vi "system to string.vi"(8 "error in":errorcluster, 11 "system":T1) -> (0 "error out":errorcluster, 2 "data":string)   [LabVIEW 2013, in "PLConfigurationSerializer.lvlib"]
uses:
  PLConfigurationSerializer.lvlib
  systems cluster.ctl
  system configuration/PL_System Configuration.lvclass
  targets cluster.ctl
  target configuration/PL_Target Configuration.lvclass
  engines cluster.ctl
  <vilib>/NI/Module Execution Interface/Engine Configuration/engine configuration.lvclass
  <vilib>/NI/Tag Bus Module Framework/module configuration/TBM module configuration.lvclass
  targetlist.ctl
  target configuration/PL_Target Configuration.lvclass/PL_Target Configuration.ctl
  enginelist.ctl
  modulelist.ctl
  <vilib>/NI/Tag Bus Module Framework/root configuration/TBM configuration.lvclass/TBM configuration.ctl
  <vilib>/NI/Tag Bus Module Framework/root configuration/create GUID.vi
  <vilib>/NI/Tag Bus Module Framework/root configuration/TBM configuration.lvclass
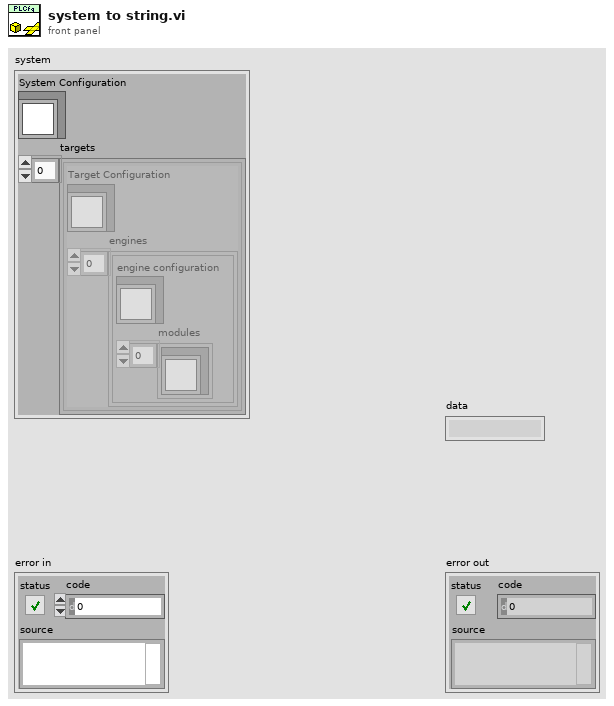
[diagram p1: front panel]
types:
  T1 = typedef "PLConfigurationSerializer.lvlib/systems cluster.ctl" = cluster{"System Configuration":refnum<class "PL_System Configuration.lvclass">, "targets":T2[]}
  T2 = typedef "PLConfigurationSerializer.lvlib/targets cluster.ctl" = cluster{"Target Configuration":refnum<class "PL_Target Configuration.lvclass">, "engines":T3[]}
  T3 = typedef "PLConfigurationSerializer.lvlib/engines cluster.ctl" = cluster{"engine configuration":refnum<class "engine configuration.lvclass">, "modules":refnum<class "TBM module configuration.lvclass">[]}
  T4 = typedef "PLConfigurationSerializer.lvlib/targetlist.ctl" = cluster{"name":string, "instanceid":string}
  T5 = typedef "PLConfigurationSerializer.lvlib/enginelist.ctl" = cluster{"engineid":string, "classname":string}
  T6 = typedef "PLConfigurationSerializer.lvlib/modulelist.ctl" = cluster{"moduleid":string, "classname":string}
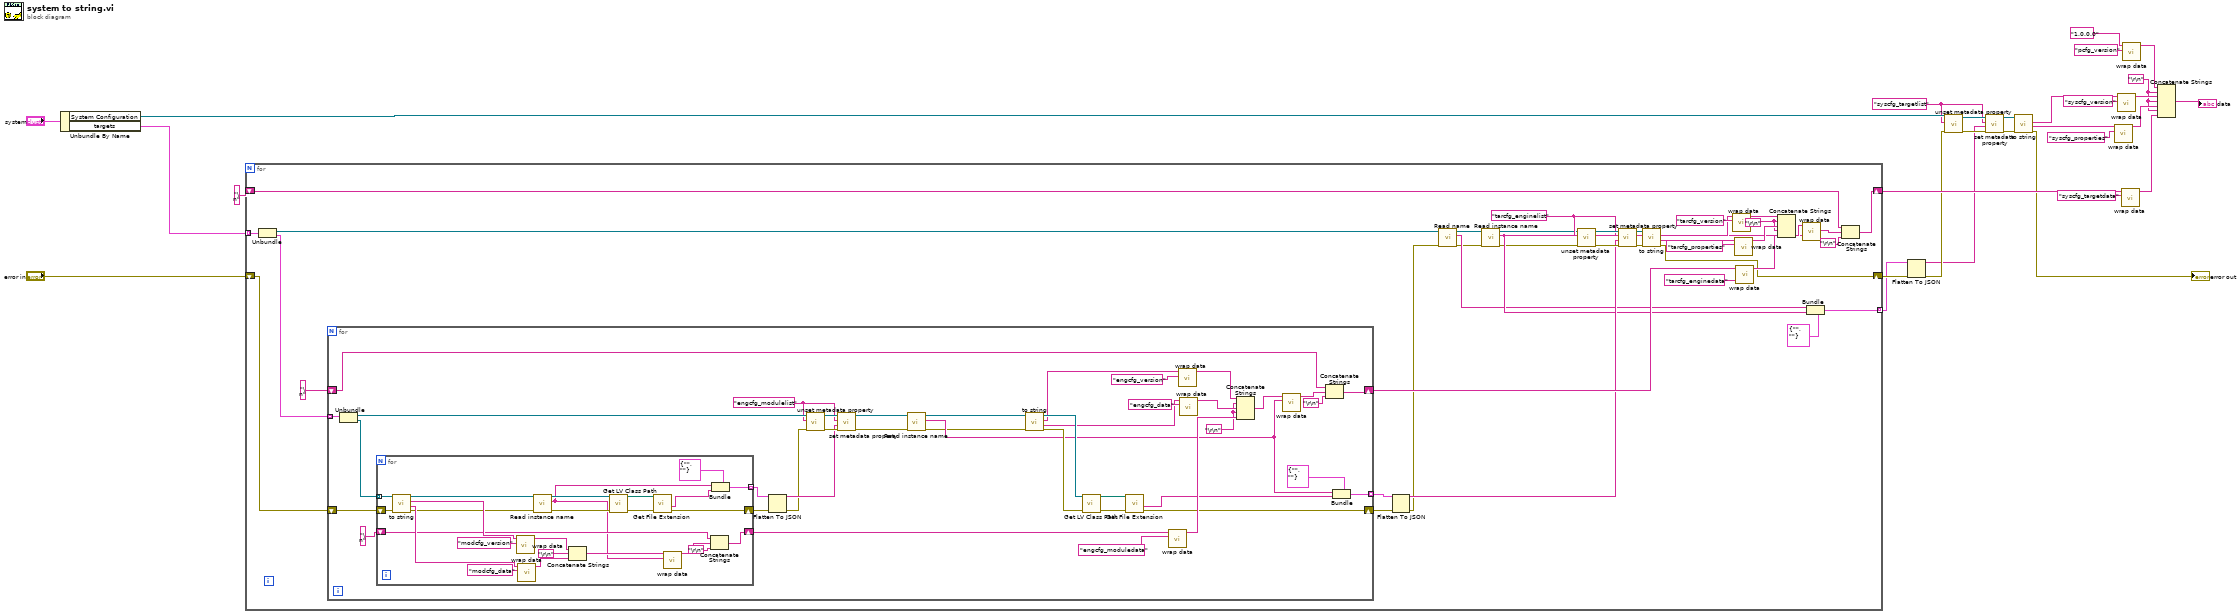
[diagram p0: block diagram]
diagram:
  w2 = "syscfg_targetlist" ("additional identifier")
  w16 = "\r\n"
  n1 = Unbundle By Name("system") -> ("System Configuration"=w7:refnum<class "PL_System Configuration.lvclass">, "targets"=w23:T2[])
  n2 = for {
    tunnel: w23 -> [w67] mode=indexing
    shift-right: [w47] -> w11
    shift-left: "error in" -> [w48]
    shift-right: [w60] -> w19
    shift-left: "\n" -> [w59]
    tunnel: [w44] -> w10 mode=indexing
    w41 = "tarcfg_enginelist" ("additional identifier")
    w52 = "\r\n"
    n3 = Unbundle(w67) -> ("Target Configuration"=w33:refnum<class "PL_Target Configuration.lvclass">, "engines"=w55:T3[])
    n4 = for {
      shift-right: [w75] -> w39
      shift-left: w48 -> [w84]
      tunnel: w55 -> [w107] mode=indexing
      shift-right: [w98] -> w50
      shift-left: "\n" -> [w97]
      tunnel: [w92] -> w40 mode=indexing
      w79 = "engcfg_modulelist" ("additional identifier")
      w87 = "\r\n"
      n5 = Unbundle(w107) -> ("engine configuration"=w80:refnum<class "engine configuration.lvclass">, "modules"=w106:refnum<class "TBM module configuration.lvclass">[])
      n6 = for {
        tunnel: w106 -> [w131] mode=indexing
        shift-right: [w111] -> w86
        shift-left: w84 -> [w132]
        shift-right: [w120] -> w100
        shift-left: "\n" -> [w118]
        tunnel: [w117] -> w83 mode=indexing
        n7 = call-dynamic "to string.vi"("error in"=w132, "module configuration in"=w131) -> ("error out"=w108:errorcluster, "data"=w127:string, "version"=w130:string, "module configuration out"=w122:refnum<class "TBM module configuration.lvclass">)  [unwired: 6 in]
        n8 = call <vilib>:"wrap data.vi"("identifier"="modcfg_version" ("additional identifier"), "data to wrap"=w130) -> ("wrapped data"=w124:string)  [unwired: 9 in]
        n9 = call <vilib>:"wrap data.vi"("identifier"="modcfg_data" ("additional identifier"), "data to wrap"=w127) -> ("wrapped data"=w126:string)  [unwired: 9 in]
        n10 = call <vilib>:"Read instance name.vi"("error in"=w108, "configuration in"=w122) -> ("error out"=w110:errorcluster, "instance id"=w109:string, "configuration out"=w112:refnum<class "TBM module configuration.lvclass">)  [unwired: 7 in]
        n11 = Concatenate Strings(w124, "\r\n", w126) -> (w123:string)
        n12 = call <vilib>:"Get LV Class Path.vi"("error in (no error)"=w110, "object"=w112) -> ("error out"=w114:errorcluster, "class path"=w115:path)  [unwired: 8 in]
        n13 = call <vilib>:"Get File Extension.vi"("error in (no error)"=w114, "file"=w115) -> ("error out"=w111:errorcluster, "filename without extension"=w113:string)  [unwired: 6 in, 2 out]
        n14 = call <vilib>:"wrap data.vi"("identifier"=w109, "data to wrap"=w123) -> ("wrapped data"=w119:string)  [unwired: 9 in]
        n15 = Concatenate Strings(w118, w119, "\r\n") -> (w120:string)
        n16 = Bundle(cluster=T6 {"moduleid"="", "classname"=""} ("modulelist"), "moduleid"=w109, "classname"=w113) -> (w117:T6)
      }
      n17 = Flatten To JSON(anything=w83, error in (no error)=w86) -> (JSON string=w78:string, 11:w77:errorcluster)  [unwired: 1 in]
      n18 = call <vilib>:"unset metadata property.vi"("error in"=w77, "key"=w79, "configuration in"=w80) -> ("error out"=w82:errorcluster, "configuration out"=w81:refnum<class "engine configuration.lvclass">)  [unwired: 7 in]
      n19 = call <vilib>:"set metadata property.vi"("error in"=w82, "value"=w78, "key"=w79, "configuration in"=w81) -> ("error out"=w68:errorcluster, "configuration out"=w69:refnum<class "engine configuration.lvclass">)  [unwired: 6 in]
      n20 = call <vilib>:"Read instance name.vi"("error in"=w68, "configuration in"=w69) -> ("error out"=w71:errorcluster, "instance id"=w72:string, "configuration out"=w70:refnum<class "engine configuration.lvclass">)  [unwired: 7 in]
      n21 = call-dynamic "to string.vi"("error in"=w71, "engine configuration in"=w70) -> ("error out"=w105:errorcluster, "data"=w93:string, "version"=w94:string, "engine configuration out"=w95:refnum<class "engine configuration.lvclass">)  [unwired: 6 in]
      n22 = call <vilib>:"Get LV Class Path.vi"("error in (no error)"=w105, "object"=w95) -> ("error out"=w76:errorcluster, "class path"=w74:path)  [unwired: 8 in]
      n23 = call <vilib>:"Get File Extension.vi"("error in (no error)"=w76, "file"=w74) -> ("error out"=w75:errorcluster, "filename without extension"=w73:string)  [unwired: 6 in, 2 out]
      n24 = call <vilib>:"wrap data.vi"("identifier"="engcfg_moduledata" ("additional identifier"), "data to wrap"=w100) -> ("wrapped data"=w89:string)  [unwired: 9 in]
      n25 = call <vilib>:"wrap data.vi"("identifier"="engcfg_version" ("additional identifier"), "data to wrap"=w94) -> ("wrapped data"=w91:string)  [unwired: 9 in]
      n26 = call <vilib>:"wrap data.vi"("identifier"="engcfg_data" ("additional identifier"), "data to wrap"=w93) -> ("wrapped data"=w90:string)  [unwired: 9 in]
      n27 = Concatenate Strings(w91, w87, w90, w87, w89) -> (w88:string)
      n28 = call <vilib>:"wrap data.vi"("identifier"=w72, "data to wrap"=w88) -> ("wrapped data"=w96:string)  [unwired: 9 in]
      n29 = Concatenate Strings(w97, w96, "\r\n") -> (w98:string)
      n30 = Bundle(cluster=T5 {"engineid"="", "classname"=""} ("enginelist"), "engineid"=w72, "classname"=w73) -> (w92:T5)
    }
    n31 = Flatten To JSON(anything=w40, error in (no error)=w39) -> (JSON string=w38:string, 11:w32:errorcluster)  [unwired: 1 in]
    n32 = call "Read name.vi"("error in"=w32, "PL_Local Target Configuration in"=w33) -> ("error out"=w31:errorcluster, "name"=w36:string, "PL_Local Target Configuration out"=w34:refnum<class "PL_Target Configuration.lvclass">)  [unwired: 7 in]
    n33 = call <vilib>:"Read instance name.vi"("error in"=w31, "configuration in"=w34) -> ("error out"=w30:errorcluster, "instance id"=w37:string, "configuration out"=w35:refnum<class "PL_Target Configuration.lvclass">)  [unwired: 7 in]
    n34 = call <vilib>:"unset metadata property.vi"("error in"=w30, "key"=w41, "configuration in"=w35) -> ("error out"=w42:errorcluster, "configuration out"=w43:refnum<class "PL_Target Configuration.lvclass">)  [unwired: 7 in]
    n35 = call <vilib>:"set metadata property.vi"("error in"=w42, "value"=w38, "key"=w41, "configuration in"=w43) -> ("error out"=w46:errorcluster, "configuration out"=w45:refnum<class "PL_Target Configuration.lvclass">)  [unwired: 6 in]
    n36 = call-dynamic "to string.vi"("error in"=w46, "configuration in"=w45) -> ("error out"=w47:errorcluster, "data"=w63:string, "version"=w65:string)  [unwired: 6 in, 1 out]
    n37 = call <vilib>:"wrap data.vi"("identifier"="tarcfg_version" ("additional identifier"), "data to wrap"=w65) -> ("wrapped data"=w62:string)  [unwired: 9 in]
    n38 = call <vilib>:"wrap data.vi"("identifier"="tarcfg_properties" ("additional identifier"), "data to wrap"=w63) -> ("wrapped data"=w61:string)  [unwired: 9 in]
    n39 = call <vilib>:"wrap data.vi"("identifier"="tarcfg_enginedata" ("additional identifier"), "data to wrap"=w50) -> ("wrapped data"=w53:string)  [unwired: 9 in]
    n40 = Concatenate Strings(w62, w52, w61, w52, w53) -> (w57:string)
    n41 = call <vilib>:"wrap data.vi"("identifier"=w37, "data to wrap"=w57) -> ("wrapped data"=w56:string)  [unwired: 9 in]
    n42 = Bundle(cluster=T4 {"name"="", "instanceid"=""} ("targetlist"), "name"=w36, "instanceid"=w37) -> (w44:T4)
    n43 = Concatenate Strings(w59, w56, "\r\n") -> (w60:string)
  }
  n44 = Flatten To JSON(anything=w10, error in (no error)=w11) -> (JSON string=w3:string, 11:w4:errorcluster)  [unwired: 1 in]
  n45 = call <vilib>:"unset metadata property.vi"("error in"=w4, "key"=w2, "configuration in"=w7) -> ("error out"=w9:errorcluster, "configuration out"=w8:refnum<class "PL_System Configuration.lvclass">)  [unwired: 7 in]
  n46 = call <vilib>:"set metadata property.vi"("error in"=w9, "value"=w3, "key"=w2, "configuration in"=w8) -> ("error out"=w5:errorcluster, "configuration out"=w6:refnum<class "PL_System Configuration.lvclass">)  [unwired: 6 in]
  n47 = call-dynamic "to string.vi"("error in"=w5, "configuration in"=w6) -> ("error out"=→"error out":errorcluster, "data"=w27:string, "version"=w29:string)  [unwired: 6 in, 1 out]
  n48 = call <vilib>:"wrap data.vi"("identifier"="syscfg_properties" ("additional identifier"), "data to wrap"=w27) -> ("wrapped data"=w24:string)  [unwired: 9 in]
  n49 = call <vilib>:"wrap data.vi"("identifier"="syscfg_version" ("additional identifier"), "data to wrap"=w29) -> ("wrapped data"=w25:string)  [unwired: 9 in]
  n50 = call <vilib>:"wrap data.vi"("identifier"="syscfg_targetdata" ("additional identifier"), "data to wrap"=w19) -> ("wrapped data"=w22:string)  [unwired: 9 in]
  n51 = call <vilib>:"wrap data.vi"("identifier"="pcfg_version" ("additional identifier"), "data to wrap"="1.0.0.0") -> ("wrapped data"=w15:string)  [unwired: 9 in]
  n52 = Concatenate Strings(w15, w16, w25, w16, w24, w16, w22) -> (→"data":string)
